vi "Normalize.vi"(11 "Vector":cluster{"X":sgl, "Y":sgl, "Z":sgl}) -> (3 "Normalized Vector":cluster{"X":sgl, "Y":sgl, "Z":sgl})   [LabVIEW 2020, in "3D Plot.lvclass"]
uses:
  3D Plot.lvclass
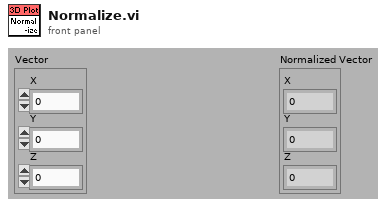
[diagram p1: front panel]
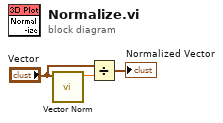
[diagram p0: block diagram]
diagram:
  n1 = call "Vector Norm.vi"("Vector"="Vector") -> ("Norm"=w1:sgl)  [unwired: 10 out]
  n2 = Divide(x="Vector", y=w1) -> (x/y=→"Normalized Vector":cluster{"X":sgl, "Y":sgl, "Z":sgl})
